vi "UpdateCOntrollerGlobal.vi"(11 "Update Frequency":dbl) -> ()   [LabVIEW 2014]
uses:
  <vilib>/Rock Robotics/WPI/Joystick/WPI_JoystickGetSetRefNum.vi
  Variables/Default global.vi
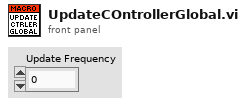
[diagram p1: front panel]
types:
  T1 = typedef "WPI_JoystickDevRef.ctl" = cluster{"Device":T2}
  T2 = typedef "WPI_JoystickDeviceEnum.ctl" = enum16{"USB 0", "USB 1", "USB 2", "USB 3", "USB 4", "USB 5"}
  T3 = cluster{"Sticks":cluster{"Left":cluster{"X":dbl, "Y":dbl, "Pressed?":bool}, "Right":cluster{"X":dbl, "Y":dbl, "Pressed?":bool}, "D-Pad":cluster{"X":dbl, "Y":dbl, "Directions":cluster{"North":bool, "Northeast":bool, "East":bool, "Southeast":bool, "South":bool, "Southwest":bool, "West":bool, "Northwest":bool}}}, "Buttons":cluster{"A":bool, "B":bool, "X":bool, "Y 3":bool, "L":bool, "R 3":bool, "Back":bool, "Start":bool}, "Triggers":cluster{"Left Trigger":cluster{"Depression":dbl, "Pressed":bool}, "Right Trigger":cluster{"Depression":dbl, "Pressed":bool}}, "Specials":cluster{"A \"SMASH\"":cluster{"Up":bool, "Down":bool, "Left":bool, "Right 3":bool}, "Double Tap":cluster{"A":bool, "B":bool, "X":bool, "Y 3":bool}, "Latching":cluster{"A":bool, "B":bool, "X":bool, "Y 3":bool, "L":bool, "R 3":bool, "Back":bool, "Start":bool}}}
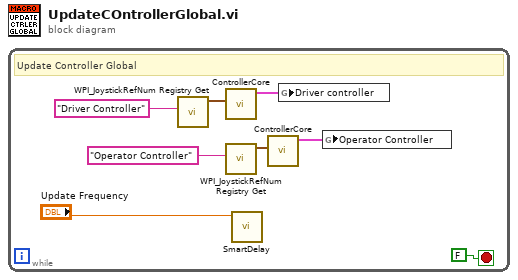
[diagram p0: block diagram]
diagram:
  n1 = while {
    stop <- FALSE stop-if-true
    # "Update Controller Global"
    n2 = call <vilib>:"WPI_JoystickRefNum Registry Get.vi"("refnum name"="Driver Controller") -> ("JoystickDevRef"=w7:T1)  [unwired: 9 in, 1 out]
    n3 = call "ControllerCore.vi"("JoystickDevRef"=w7) -> ("Driver controller"=w6:T3)  [unwired: 9 in, 1 out]
    n4 = call <vilib>:"WPI_JoystickRefNum Registry Get.vi"("refnum name"="Operator Controller") -> ("JoystickDevRef"=w4:T1)  [unwired: 9 in, 1 out]
    n5 = call "SmartDelay.vi"("Frequency"="Update Frequency") -> ()  [unwired: 11 in]
    n6 = call "ControllerCore.vi"("JoystickDevRef"=w4) -> ("Driver controller"=w5:T3)  [unwired: 9 in, 1 out]
    n7 = global write "Default global.vi" "Driver controller"(w6) -> ()
    n8 = global write "Default global.vi" "Operator Controller"(w5) -> ()
  }
